vi "VI_Synchronization.vi"() -> ()   [LabVIEW 2022 SP3]
uses:
  <vilib>/Utility/error.llb/DialogType.ctl
  <vilib>/DAQmx/read.llb/DAQmx Read (Analog Wfm 1Chan NSamp).vi
  <vilib>/DAQmx/create/channels.llb/DAQmx Create Channel (AI-Force-Bridge-Two-Point-Linear).vi
  <vilib>/DAQmx/configure/timing.llb/DAQmx Timing (Sample Clock).vi
  <vilib>/DAQmx/create/channels.llb/DAQmx Create Channel (AI-Voltage-Basic).vi
  <vilib>/DAQmx/configure/trigger.llb/DAQmx Start Trigger (Digital Edge).vi
  <vilib>/DAQmx/miscellaneous.llb/DAQmx Fill In Error Info.vi
  <resource>/objmgr/daqmx.rc
panel:
  in  "stop":bool
  out "Waveform Chart 2":waveform(dbl)(graph)
  out "Waveform Chart":waveform(dbl)(graph)
  in  "error in 3":errorcluster caption="error in"
  in  "error in":errorcluster
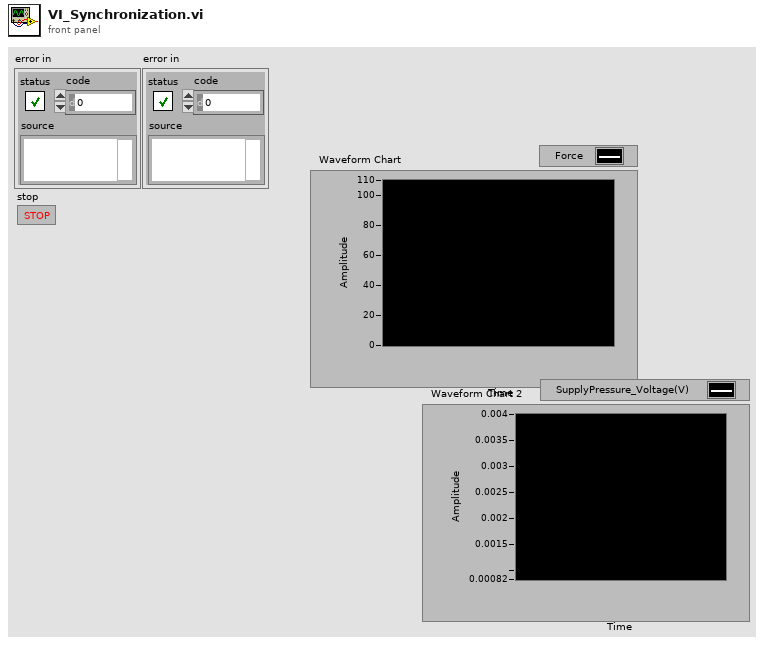
[diagram p1: front panel]
types:
  T1 = typedef "DialogType.ctl" = u16
  T2 = cluster{"first electrical value":dbl, "second electrical value":dbl, "electrical units":i32, "first physical value":dbl, "second physical value":dbl, "physical units":i32}
  T3 = cluster{"bridge configuration":i32, "voltage excitation source":i32, "voltage excitation value":dbl, "nominal bridge resistance":dbl}
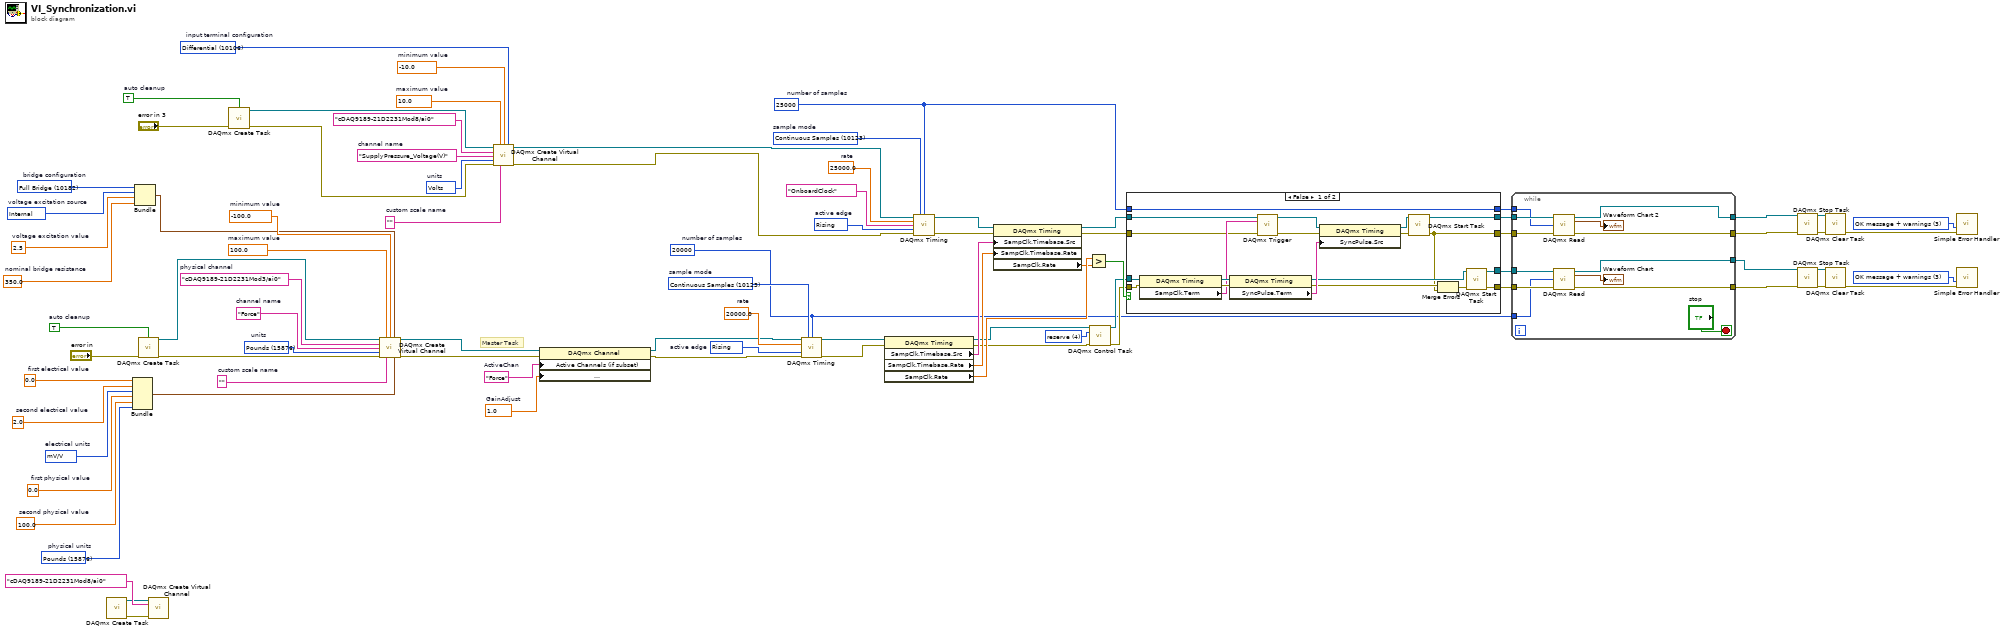
[diagram p0: block diagram]
diagram:
  w10 = T1 3 items=["no dialog", "OK message", "continue or stop message", "OK message + warnings", "continue/stop + warnings"] ("type of dialog (OK msg:1)")
  w7 = T1 3 items=["no dialog", "OK message", "continue or stop message", "OK message + warnings", "continue/stop + warnings"] ("type of dialog (OK msg:1)")
  w28 = 4 items=["verify"=2, "reserve"=4, "commit"=3, "unreserve"=5, "abort"=6] ("action")
  w45 = 10123 items=["Finite Samples"=10178, "Continuous Samples"=10123, "Hardware Timed Single Point"=12522]  # sample mode
  w46 = 25000.0  # rate
  w47 = 10280 items=["Rising"=10280, "Falling"=10171]  # active edge
  w17 = 25000  # number of samples
  w48 = 10106 items=["default"=-1, "RSE"=10083, "NRSE"=10078, "Differential"=10106, "Pseudodifferential"=12529]  # input terminal configuration
  w49 = 10348 items=["Volts"=10348, "From Custom Scale"=10065]  # units
  w50 = "SupplyPressure_Voltage(V)"  # channel name
  w51 = ""  # custom scale name
  w52 = -10.0  # minimum value
  w53 = 10.0  # maximum value
  w55 = TRUE  # auto cleanup
  w58 = 10123 items=["Finite Samples"=10178, "Continuous Samples"=10123, "Hardware Timed Single Point"=12522]  # sample mode
  w59 = 20000.0  # rate
  w60 = 10280 items=["Rising"=10280, "Falling"=10171]  # active edge
  w21 = 20000  # number of samples
  w61 = 1.0  # GainAdjust
  w63 = "Force"  # ActiveChan
  w64 = 15876 items=["Newtons"=15875, "Pounds"=15876, "kgf"=15877]  # physical units
  w70 = 0.0  # first electrical value
  w69 = 2.0  # second electrical value
  w68 = 15897 items=["V/V"=15896, "mV/V"=15897]  # electrical units
  w67 = 0.0  # first physical value
  w66 = 100.0  # second physical value
  w72 = 350.0  # nominal bridge resistance
  w73 = 2.5  # voltage excitation value
  w74 = 10200 items=["Internal"=10200, "External"=10167]  # voltage excitation source
  w75 = 10182 items=["Full Bridge"=10182, "Half Bridge"=10187, "Quarter Bridge"=10270]  # bridge configuration
  w76 = 15876 items=["Newtons"=15875, "Pounds"=15876, "kgf"=15877, "From Custom Scale"=10065]  # units
  w77 = "Force"  # channel name
  w79 = ""  # custom scale name
  w80 = -100.0  # minimum value
  w81 = 100.0  # maximum value
  w82 = "cDAQ9189-21D2231Mod3/ai0"  # physical channel
  w84 = TRUE  # auto cleanup
  # "Master Task"
  n1 = call <vilib>:"DAQmx Create Task.vi"() -> ("task out"=w42:refnum<k21>, "error out"=w41:errorcluster)  [unwired: 14 in]
  n2 = Bundle("first electrical value"=w70, "second electrical value"=w69, "electrical units"=w68, "first physical value"=w67, "second physical value"=w66, "physical units"=w64) -> (w65:T2)  [unwired: 1 in]
  n3 = Bundle("bridge configuration"=w75, "voltage excitation source"=w74, "voltage excitation value"=w73, "nominal bridge resistance"=w72) -> (w71:T3)  [unwired: 1 in]
  n4 = call <vilib>:"DAQmx Create Task.vi"("auto cleanup"=w84, "error in"="error in") -> ("task out"=w83:refnum<k21>, "error out"=w85:errorcluster)  [unwired: 12 in]
  n5 = call-poly <vilib>:"DAQmx Create Virtual Channel.vi"("task in"=w42, "physical channels"=tag "cDAQ9189-21D2231Mod8/ai0", "error in"=w41) -> ()  [unwired: 11 in, 2 out]
  n6 = call <vilib>:"DAQmx Create Task.vi"("auto cleanup"=w55, "error in"="error in 3") -> ("task out"=w54:refnum<k21>, "error out"=w56:errorcluster)  [unwired: 12 in]
  n7 = call-poly <vilib>:"DAQmx Create Virtual Channel.vi"("task in"=w83, "maximum value"=w81, "minimum value"=w80, "bridge information"=w71, "physical channels"=w82, "name to assign"=w77, "units"=w76, "error in"=w85, "custom scale name"=w79, "scaling information"=w65) -> ("task out"=w62:refnum<k21>, "error out"=w78:errorcluster)  [unwired: 4 in]
  n8 = call-poly <vilib>:"DAQmx Create Virtual Channel.vi"("task in"=w54, "maximum value"=w53, "minimum value"=w52, "input terminal configuration"=w48, "physical channels"=tag "cDAQ9189-21D2231Mod8/ai0", "name to assign"=w50, "units"=w49, "error in"=w56, "custom scale name"=w51) -> ("task out"=w1:refnum<k21>, "error out"=w2:errorcluster)  [unwired: 5 in]
  n9 = property class="DAQmx Channel"(reference=w62, error in=w78, "Active Channels (if subset)"=w63, "Analog Input:General Properties:Signal Conditioning:Bridge:Shunt Cal:Gain Adjustment"=w61) -> (reference out=w4:refnum<k21>, error out=w3:errorcluster)
  n10 = call-poly <vilib>:"DAQmx Timing.vi"("task/channels in"=w4, "sample mode"=w58, "samples per channel"=w21, "rate"=w59, "active edge"=w60, "error in"=w3) -> ("task out"=w38:refnum<k21>, "error out"=w39:errorcluster)  [unwired: 8 in]
  n11 = property class="DAQmx Timing"(reference=w38, error in=w39) -> (reference out=w30:refnum<k21>, error out=w29:errorcluster, "SampClk.Timebase.Src"=w35:tag, "SampClk.Timebase.Rate"=w34:dbl, "SampClk.Rate"=w33:dbl)
  n12 = call-poly <vilib>:"DAQmx Timing.vi"("task/channels in"=w1, "sample mode"=w45, "samples per channel"=w17, "rate"=w46, "source"=tag "OnboardClock", "active edge"=w47, "error in"=w2) -> ("task out"=w37:refnum<k21>, "error out"=w36:errorcluster)  [unwired: 7 in]
  n13 = property class="DAQmx Timing"(reference=w37, error in=w36, "SampClk.Timebase.Src"=w35, "SampClk.Timebase.Rate"=w34) -> (reference out=w25:refnum<k21>, error out=w24:errorcluster, "SampClk.Rate"=w32:dbl)
  n14 = Greater?(x=w33, y=w32) -> (0:w31:bool)
  n15 = call <vilib>:"DAQmx Control Task.vi"("task/channels in"=w30, "action"=w28, "error in"=w29) -> ("task out"=w27:refnum<k21>, "error out"=w26:errorcluster)  [unwired: 11 in]
  n16 = case shown="False" w31 {
    tunnel: w27 -> [w106 w111]
    tunnel: w26 -> [w105 w110]
    tunnel: w25 -> [w102 w109]
    tunnel: w24 -> [w100 w108]
    tunnel: [w91 w111] -> w23
    tunnel: [w90 w110] -> w22
    tunnel: [w89 w109] -> w20
    tunnel: [w88 w108] -> w19
    tunnel: [w87 w107] -> w18
    tunnel: w17 -> [w87 w107]
    frame False {
      n17 = property class="DAQmx Timing"(reference=w106, error in=w105) -> (reference out=w104:refnum<k21>, error out=w103:errorcluster, "SampClk.Term"=w101:tag)
      n18 = property class="DAQmx Timing"(reference=w104, error in=w103) -> (reference out=w92:refnum<k21>, error out=w94:errorcluster, "SyncPulse.Term"=w97:tag)
      n19 = call-poly <vilib>:"DAQmx Trigger.vi"("task/channels in"=w102, "source"=w101, "error in"=w100) -> ("task out"=w99:refnum<k21>, "error out"=w98:errorcluster)  [unwired: 11 in]
      n20 = property class="DAQmx Timing"(reference=w99, error in=w98, "SyncPulse.Src"=w97) -> (reference out=w95:refnum<k21>, error out=w96:errorcluster)
      n21 = call <vilib>:"DAQmx Start Task.vi"("task/channels in"=w95, "error in"=w96) -> ("task out"=w89:refnum<k21>, "error out"=w88:errorcluster)  [unwired: 12 in]
      n22 = Merge Errors(w94, w88) -> (w93:errorcluster)
      n23 = call <vilib>:"DAQmx Start Task.vi"("task/channels in"=w92, "error in"=w93) -> ("task out"=w91:refnum<k21>, "error out"=w90:errorcluster)  [unwired: 12 in]
    }
    frame True {
    }
  }
  n24 = while {
    tunnel: w23 -> [w124]
    tunnel: w22 -> [w123]
    tunnel: w21 -> [w122]
    tunnel: w20 -> [w121]
    tunnel: w19 -> [w120]
    tunnel: w18 -> [w119]
    tunnel: [w115] -> w9
    tunnel: [w114] -> w8
    tunnel: [w113] -> w6
    tunnel: [w112] -> w5
    stop <- "stop" stop-if-true
    n25 = call-poly <vilib>:"DAQmx Read.vi"("task/channels in"=w121, "number of samples per channel"=w119, "error in"=w120) -> ("task out"=w115:refnum<k21>, "data"=→"Waveform Chart 2":waveform(dbl), "error out"=w114:errorcluster)  [unwired: 10 in]
    n26 = call-poly <vilib>:"DAQmx Read.vi"("task/channels in"=w124, "number of samples per channel"=w122, "error in"=w123) -> ("task out"=w113:refnum<k21>, "data"=→"Waveform Chart":waveform(dbl), "error out"=w112:errorcluster)  [unwired: 10 in]
  }
  n27 = call <vilib>:"DAQmx Stop Task.vi"("task/channels in"=w9, "error in"=w8) -> ("task out"=w15:refnum<k21>, "error out"=w14:errorcluster)  [unwired: 12 in]
  n28 = call <vilib>:"DAQmx Stop Task.vi"("task/channels in"=w6, "error in"=w5) -> ("task out"=w12:refnum<k21>, "error out"=w11:errorcluster)  [unwired: 12 in]
  n29 = call <vilib>:"DAQmx Clear Task.vi"("task in"=w15, "error in"=w14) -> ("error out"=w16:errorcluster)  [unwired: 13 in]
  n30 = call <vilib>:"DAQmx Clear Task.vi"("task in"=w12, "error in"=w11) -> ("error out"=w13:errorcluster)  [unwired: 13 in]
  n31 = call <vilib>:"Simple Error Handler.vi"("type of dialog (OK msg:1)"=w10, "error in (no error)"=w16) -> ()  [unwired: 3 in, 5 out]
  n32 = call <vilib>:"Simple Error Handler.vi"("type of dialog (OK msg:1)"=w7, "error in (no error)"=w13) -> ()  [unwired: 3 in, 5 out]
